vi "Initialize.vi"(7 "not in use":string="Setpoint.ch%d.SP", 8 "error in":errorcluster, 9 "Number of Channels":u32=1, 10 "Instance Name":string, 11 "ExampleDevice in":refnum<class "Example Device.lvclass">) -> (0 "error out":errorcluster, 3 "ExampleDevice out":refnum<class "Example Device.lvclass">)   [LabVIEW 2023, in "Example Device.lvclass"]
uses:
  Example Device.lvclass
  Example Device.lvclass/Example Device.ctl
  Current Setpoint/Current Setpoint.lvclass
  Voltage Setpoint/Voltage Setpoint.lvclass
  Current Actual Value/Current Actual Value.lvclass
  Voltage Actual Value/Voltage Actual Value.lvclass
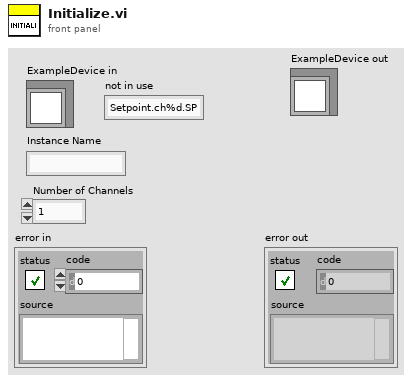
[diagram p1: front panel]
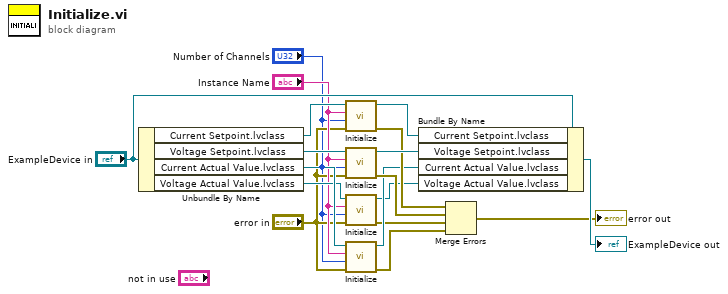
[diagram p0: block diagram]
diagram:
  n1 = Unbundle By Name("ExampleDevice in") -> ("Current Setpoint.lvclass"=w18:refnum<class "Current Setpoint.lvclass">, "Voltage Setpoint.lvclass"=w17:refnum<class "Voltage Setpoint.lvclass">, "Current Actual Value.lvclass"=w9:refnum<class "Current Actual Value.lvclass">, "Voltage Actual Value.lvclass"=w8:refnum<class "Voltage Actual Value.lvclass">)
  n2 = call-dynamic "Initialize.vi"("error in"="error in", "Number of Channels"="Number of Channels", "Instance Name"="Instance Name", "Current Setpoint in"=w18) -> ("error out 2"=w11:errorcluster, "Current Setpoint out"=w16:refnum<class "Current Setpoint.lvclass">)  [unwired: 6 in]
  n3 = call-dynamic "Initialize.vi"("error in"="error in", "Number of Channels"="Number of Channels", "Instance Name"="Instance Name", "Voltage Setpoint in"=w17) -> ("error out 2"=w12:errorcluster, "Voltage Setpoint out"=w15:refnum<class "Voltage Setpoint.lvclass">)  [unwired: 6 in]
  n4 = call-dynamic "Initialize.vi"("error in"="error in", "Number of Channels"="Number of Channels", "Instance Name"="Instance Name", "Voltage Actual Value in"=w8) -> ("error out"=w2:errorcluster, "Voltage Actual Value out"=w6:refnum<class "Voltage Actual Value.lvclass">)  [unwired: 6 in]
  n5 = call-dynamic "Initialize.vi"("error in"="error in", "Number of Channels"="Number of Channels", "Instance Name"="Instance Name", "Current Actual Value in"=w9) -> ("error out"=w1:errorcluster, "Current Actual Value out"=w7:refnum<class "Current Actual Value.lvclass">)  [unwired: 6 in]
  n6 = Bundle By Name(cluster="ExampleDevice in", "Current Setpoint.lvclass"=w16, "Voltage Setpoint.lvclass"=w15, "Current Actual Value.lvclass"=w7, "Voltage Actual Value.lvclass"=w6) -> (→"ExampleDevice out":refnum<class "Example Device.lvclass">)
  n7 = Merge Errors(w11, w12, w2, w1) -> (→"error out":errorcluster)
